vi "FPGA (POT TEST).vi"() -> ()   [LabVIEW 2017]
uses:
  <vilib>/rvi/Emulation/niFpgaGetClockAttributes.vi
  <vilib>/rvi/Emulation/niFpgaSctlEmulationGetInTimedLoop.vi
  <vilib>/rvi/Emulation/niFpgaEmulationReportErrorSimple.vi
  <vilib>/rvi/eio/common/nirviEmuTemplateMethod_errors.vi
  <vilib>/rvi/Emulation/niFpgaCriticalErrorInLSC.vi
  <vilib>/eio/EIONode/EIONode.xnode
panel:
  out "AI2_RAW":u16
  out "AI1_RAW":u16
  out "POT2_POS":u16
  out "POT1_POS":u16
  in  "LINK2_OFFSET":i16
  in  "LINK2_POT_SCALE":i16
  in  "LINK1_OFFSET":i16
  in  "LINK1_POT_SCALE":i16
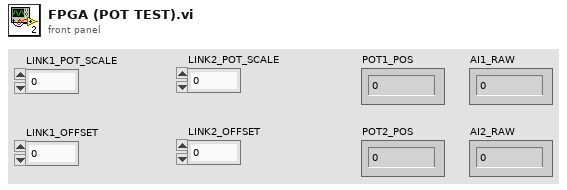
[diagram p1: front panel]
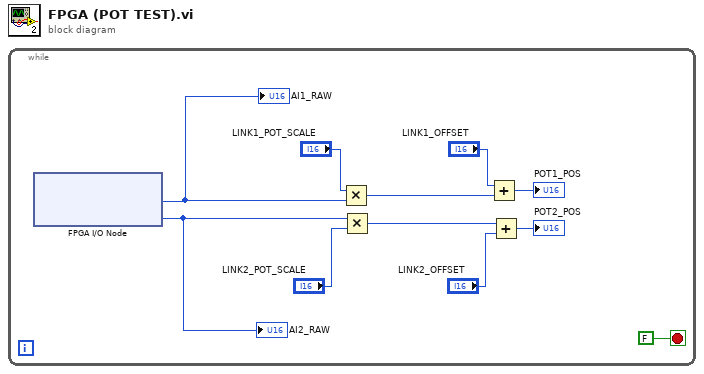
[diagram p0: block diagram]
diagram:
  n1 = while {
    stop <- FALSE stop-if-true
    n2 = xnode "FPGA I/O Node"() -> ("ConnectorB/AI1"=w10:u16, "ConnectorB/AI2"=w4:u16)  [unwired: 2 in, 2 out]
    "AI1_RAW" <- w10
    "AI2_RAW" <- w4
    n3 = Multiply(x="LINK1_POT_SCALE", y=w10) -> (x*y=w8:u16)
    n4 = Multiply(x=w4, y="LINK2_POT_SCALE") -> (x*y=w3:u16)
    n5 = Add(x="LINK1_OFFSET", y=w8) -> (x+y=→"POT1_POS":u16)
    n6 = Add(x=w3, y="LINK2_OFFSET") -> (x+y=→"POT2_POS":u16)
  }
